vi "자판기 만들기 실습.vi"() -> ()   [LabVIEW 2020]
panel:
  in  "정지":bool
  in  "거스름돈 반환":bool
  out "배출 상품명":string
  out "현재잔액":dbl
  in  "1000원":bool
  in  "500원":bool
  in  "100원":bool
  in  "50원":bool
  in  "10원":bool
  out "웰치스 LED":bool
  out "콜라 LED":bool
  out "환타 LED":bool
  out "사이다 LED":bool
  in  "웰치스":bool
  in  "콜라":bool
  in  "환타":bool
  in  "사이다":bool
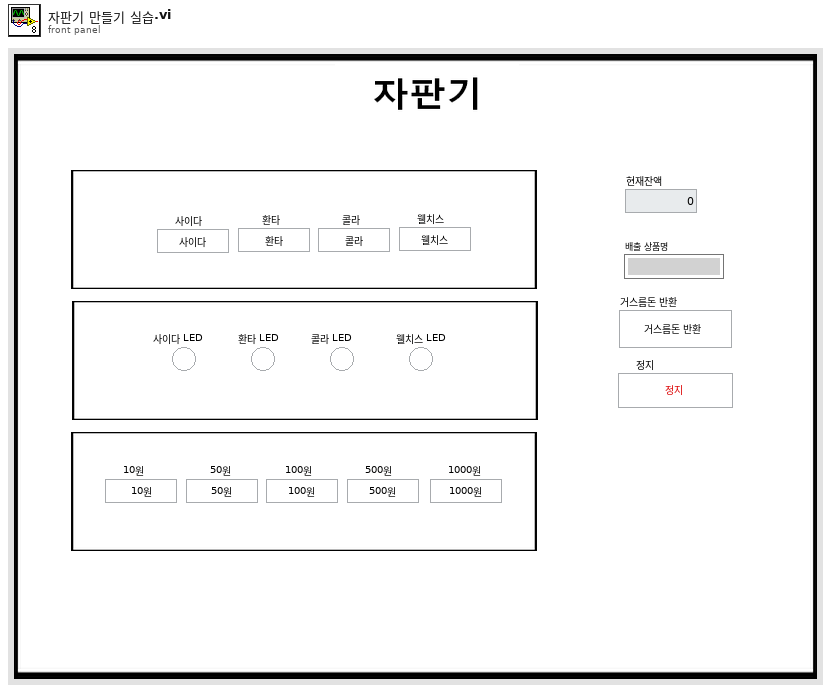
[diagram p1: front panel]
types:
  T1 = typedef "자판기 컨트롤.ctl" = enum16{"초기화", "대기", "10원", "50원", "100원", "500원", "1000원", "디스플레이 업데이트", "사이다", "콜라", "환타", "웰치스", "거스름돈 반환", "종료"}
  T2 = cluster{"상태":T1, "사이다 LED":bool, "현재잔액":dbl, "웰치스 LED":bool, "환타 LED":bool, "콜라 LED":bool, "배출 상품명":string}
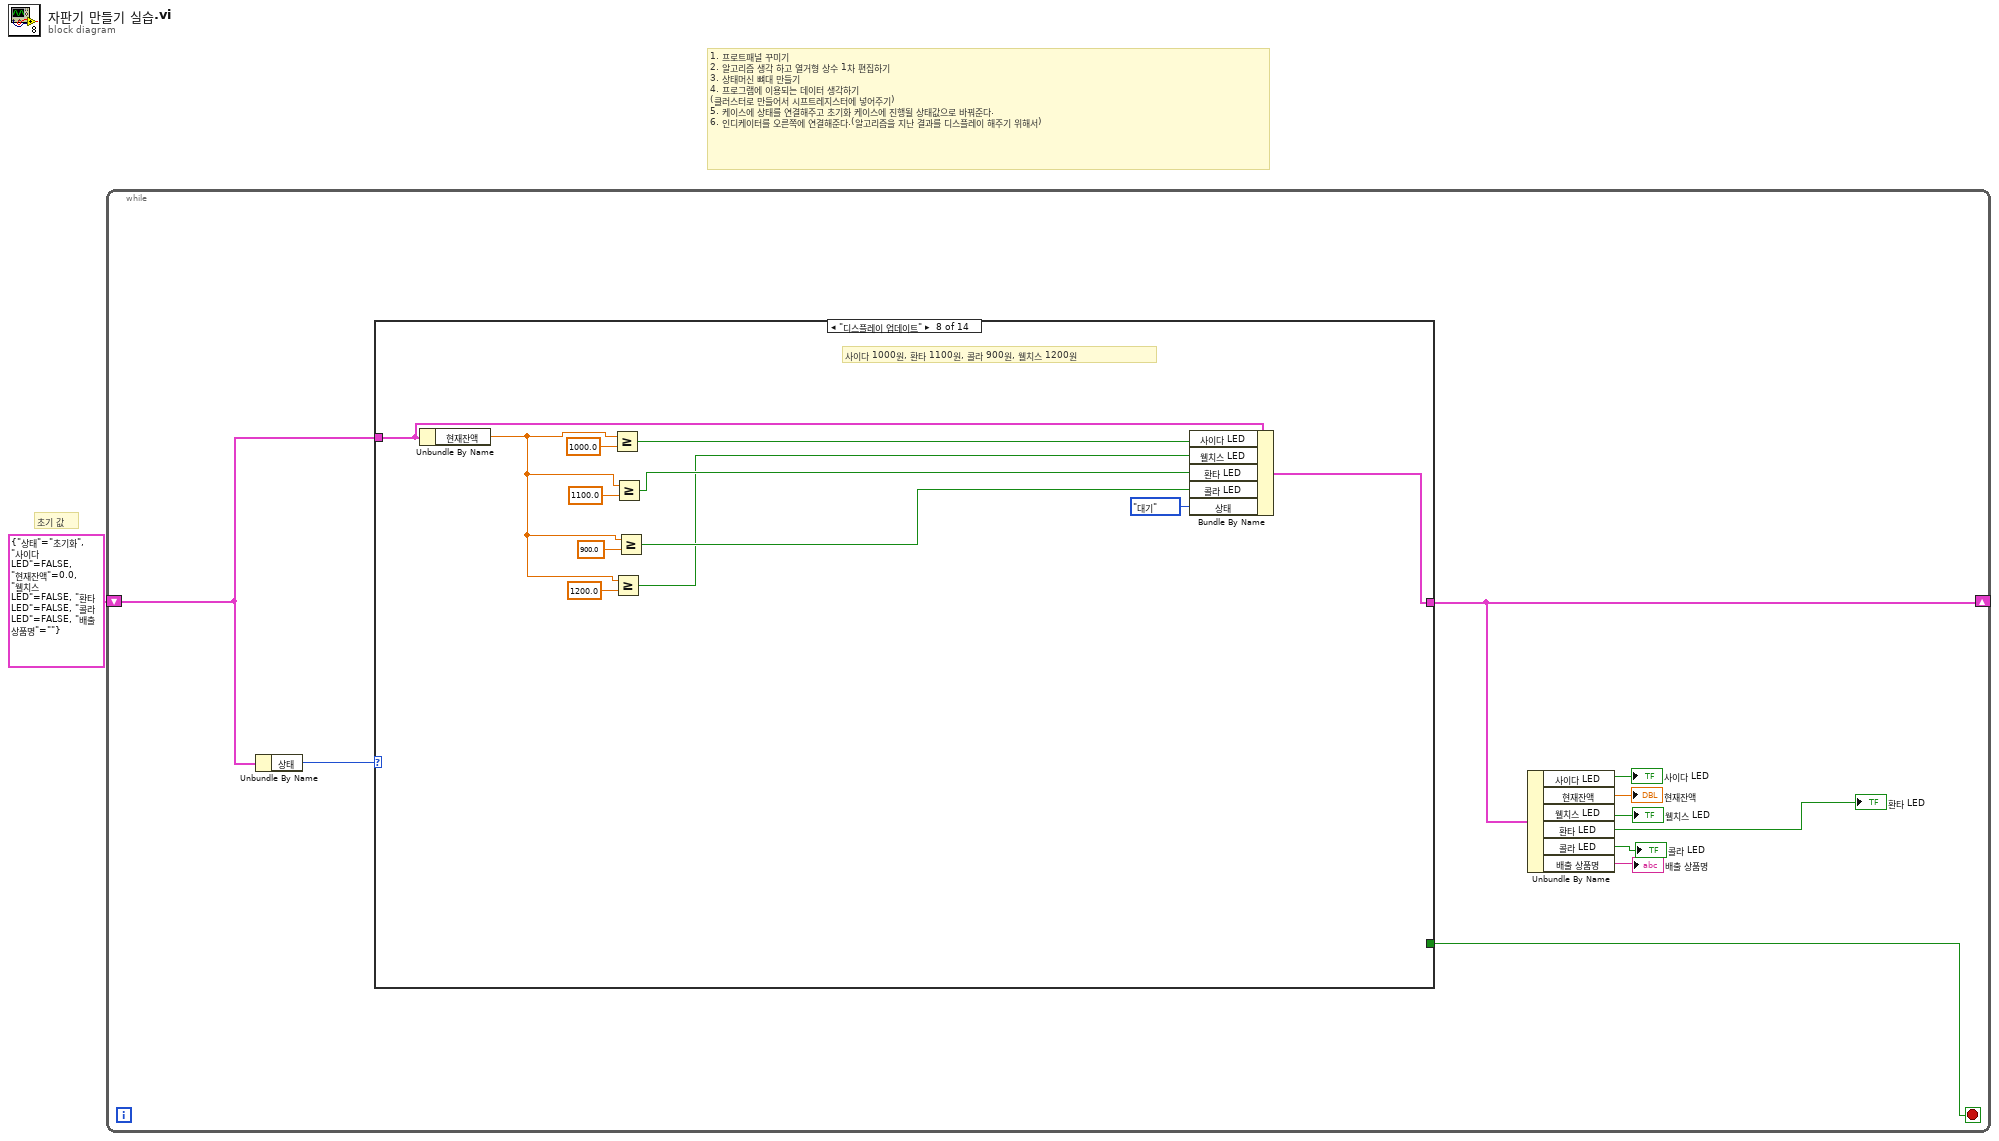
[diagram p0: block diagram]
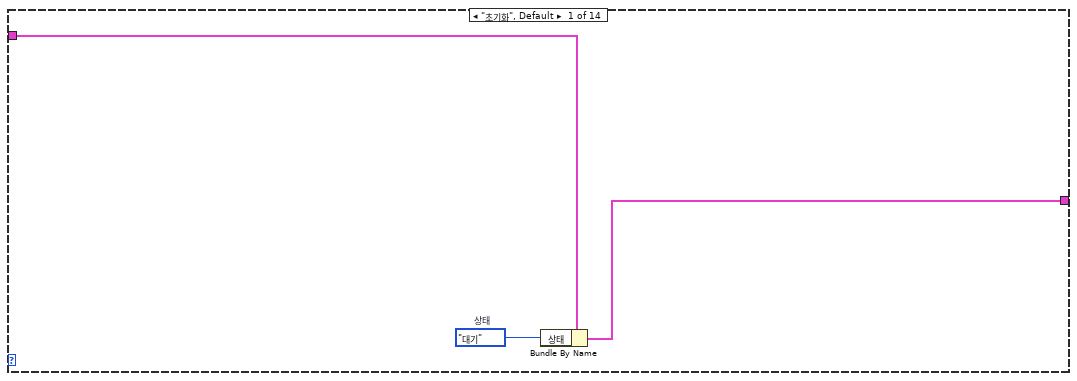
[diagram p2: hidden frame]
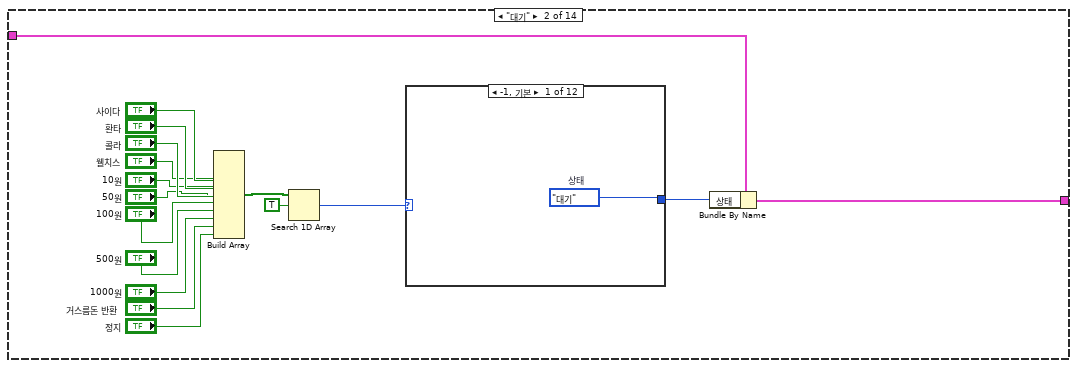
[diagram p3: hidden frame]
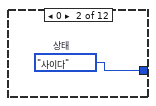
[diagram p4: hidden frame]
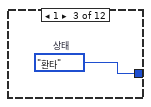
[diagram p5: hidden frame]
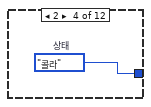
[diagram p6: hidden frame]
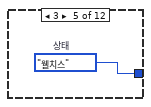
[diagram p7: hidden frame]
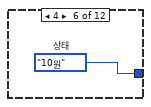
[diagram p8: hidden frame]
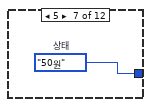
[diagram p9: hidden frame]
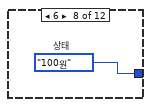
[diagram p10: hidden frame]
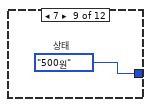
[diagram p11: hidden frame]
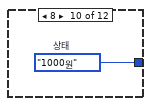
[diagram p12: hidden frame]
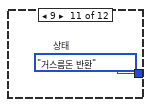
[diagram p13: hidden frame]
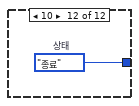
[diagram p14: hidden frame]
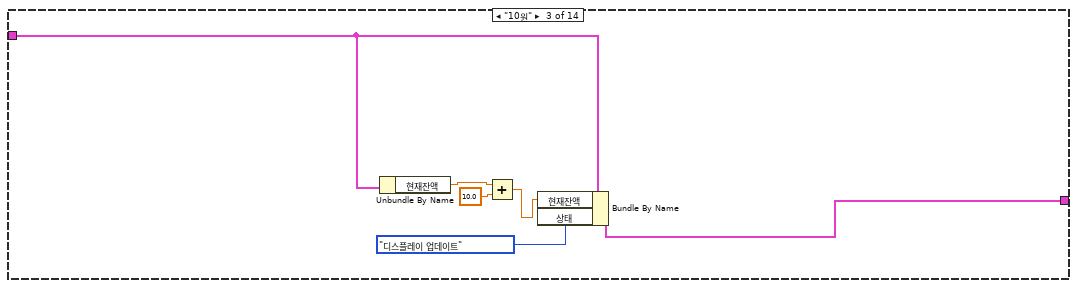
[diagram p15: hidden frame]
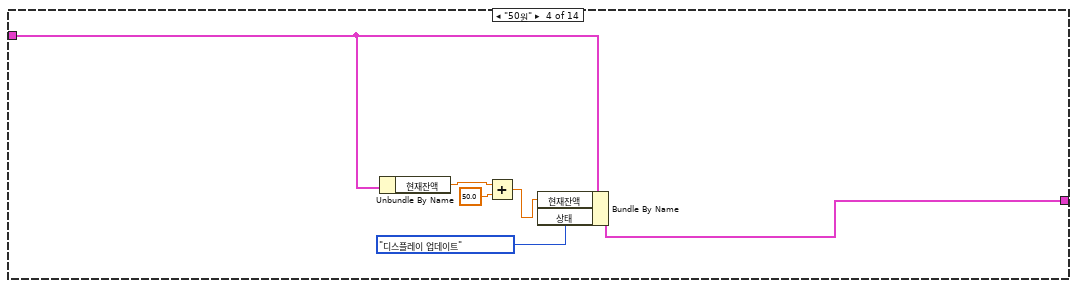
[diagram p16: hidden frame]
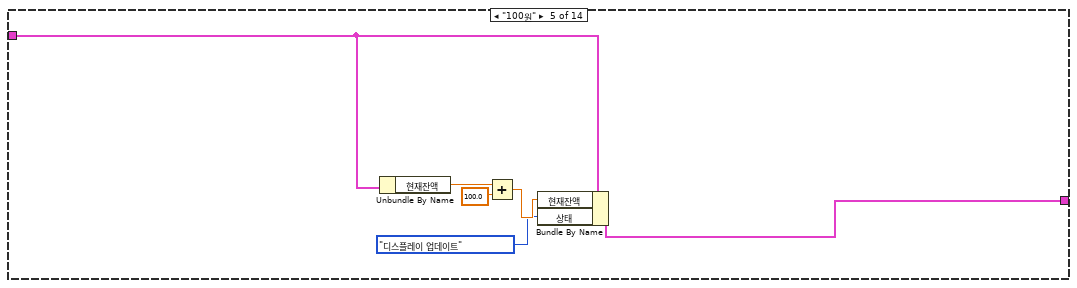
[diagram p17: hidden frame]
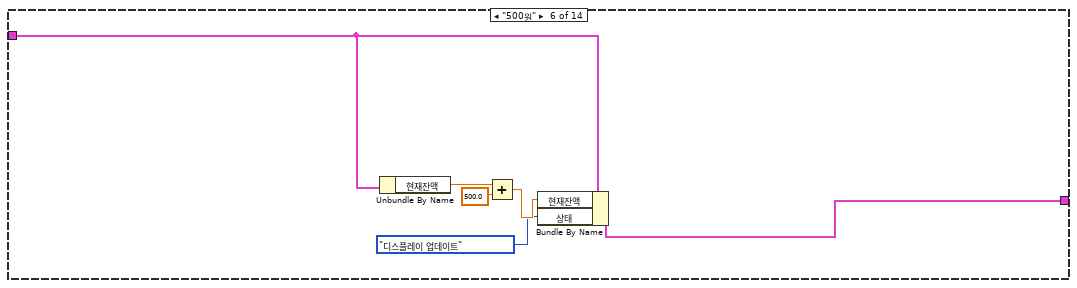
[diagram p18: hidden frame]
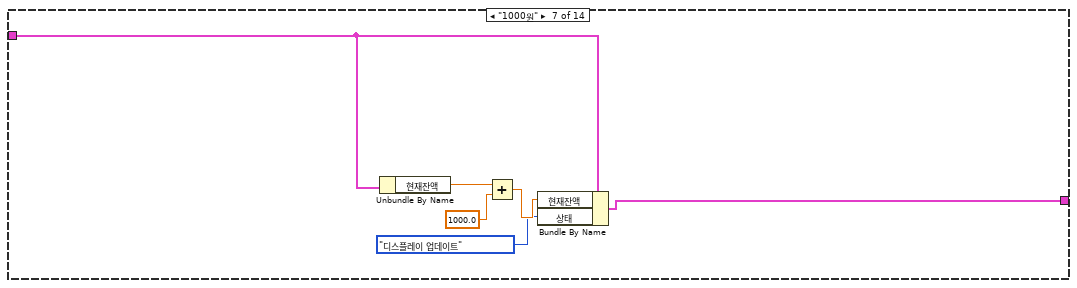
[diagram p19: hidden frame]
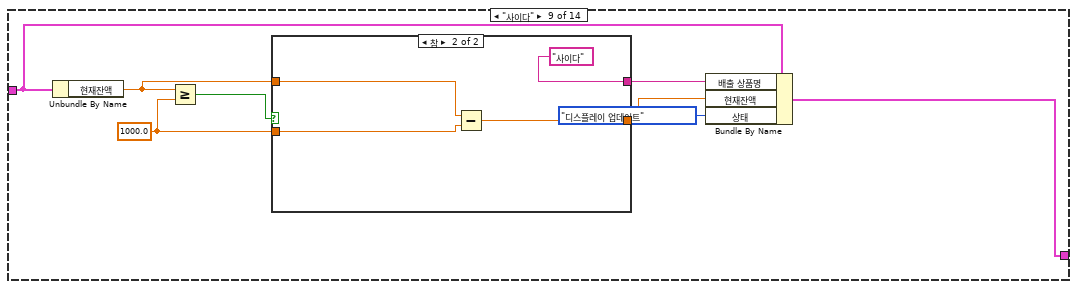
[diagram p20: hidden frame]
diagram:
  # "초기 값"
  # "1. 프로트패널 꾸미기\n2. 알고리즘 생각 하고 열거형 상수 1차 편집하기\n3. 상태머신 뼈대 만들기\n4. 프로그램에 이용되는 데이터 생각하기\n(클러스터로 만들어서 시프트레지스터에 넣어주기)\n5. 케이스에 상태를 연결해주고 초기화 케이스에 진행될 상태값으로 바꿔준다.\n6. 인디케이터를 오른쪽에 연결해준다.(알고리즘을 지난 결과를 디스플레이 해주기 위해서)"
  n1 = while {
    shift-right: [w9] -> _
    shift-left: T2 {"상태"=enum."초기화", "사이다 LED"=FALSE, "현재잔액"=0.0, "웰치스 LED"=FALSE, "환타 LED"=FALSE, "콜라 LED"=FALSE, "배출 상품명"=""} -> [w10]
    stop <- w5 stop-if-true
    n2 = Unbundle By Name(w10) -> ("상태"=w11:T1)
    n3 = case shown="\"디스플레이 업데이트\"" w11 {
      tunnel: w10 -> [w14 w17 w47 w53 w59 w65 w71 w84 w92 w106 w120 w134 w146 _]
      tunnel: [w12 w16 w45 w51 w57 w63 w69 w75 w90 w104 w118 w132 w145 _] -> w9
      tunnel: [_ _ _ _ _ _ _ _ _ _ _ _ _ TRUE] -> w5
      frame "초기화", Default {
        w13 = 자판기_컨트롤."대기"  # 상태
        n4 = Bundle By Name(cluster=w14, "상태"=w13) -> (w12:T2)
      }
      frame "대기" {
        n5 = Build Array("사이다", "환타", "콜라", "웰치스", "10원", "50원", "100원", "500원", "1000원", "거스름돈 반환", "정지") -> (w20:bool[])
        n6 = Search 1D Array(1D array=w20, element=TRUE ("원소")) -> (index of element=w18:i32)  [unwired: 1 in]
        n7 = case shown="-1, 기본" w18 {
          tunnel: [w32 w33 w34 w35 w36 w37 w38 w39 w40 w41 w42 w43] -> w15
          frame -1, Default {
            w32 = 자판기_컨트롤."대기"  # 상태
          }
          frame 0 {
            w33 = 자판기_컨트롤."사이다"  # 상태
          }
          frame 1 {
            w34 = 자판기_컨트롤."환타"  # 상태
          }
          frame 2 {
            w35 = 자판기_컨트롤."콜라"  # 상태
          }
          frame 3 {
            w36 = 자판기_컨트롤."웰치스"  # 상태
          }
          frame 4 {
            w37 = 자판기_컨트롤."10원"  # 상태
          }
          frame 5 {
            w38 = 자판기_컨트롤."50원"  # 상태
          }
          frame 6 {
            w39 = 자판기_컨트롤."100원"  # 상태
          }
          frame 7 {
            w40 = 자판기_컨트롤."500원"  # 상태
          }
          frame 8 {
            w41 = 자판기_컨트롤."1000원"  # 상태
          }
          frame 9 {
            w42 = 자판기_컨트롤."거스름돈 반환"  # 상태
          }
          frame 10 {
            w43 = 자판기_컨트롤."종료"  # 상태
          }
        }
        n8 = Bundle By Name(cluster=w17, "상태"=w15) -> (w16:T2)
      }
      frame "10원" {
        n9 = Unbundle By Name(w47) -> ("현재잔액"=w49:dbl)
        n10 = Add(x=w49, y=10.0) -> (x+y=w46:dbl)
        n11 = Bundle By Name(cluster=w47, "현재잔액"=w46, "상태"=자판기_컨트롤."디스플레이 업데이트") -> (w45:T2)
      }
      frame "50원" {
        n12 = Unbundle By Name(w53) -> ("현재잔액"=w55:dbl)
        n13 = Add(x=w55, y=50.0) -> (x+y=w52:dbl)
        n14 = Bundle By Name(cluster=w53, "현재잔액"=w52, "상태"=자판기_컨트롤."디스플레이 업데이트") -> (w51:T2)
      }
      frame "100원" {
        n15 = Unbundle By Name(w59) -> ("현재잔액"=w61:dbl)
        n16 = Add(x=w61, y=100.0) -> (x+y=w58:dbl)
        n17 = Bundle By Name(cluster=w59, "현재잔액"=w58, "상태"=자판기_컨트롤."디스플레이 업데이트") -> (w57:T2)
      }
      frame "500원" {
        n18 = Unbundle By Name(w65) -> ("현재잔액"=w67:dbl)
        n19 = Add(x=w67, y=500.0) -> (x+y=w64:dbl)
        n20 = Bundle By Name(cluster=w65, "현재잔액"=w64, "상태"=자판기_컨트롤."디스플레이 업데이트") -> (w63:T2)
      }
      frame "1000원" {
        n21 = Unbundle By Name(w71) -> ("현재잔액"=w73:dbl)
        n22 = Add(x=w73, y=1000.0) -> (x+y=w70:dbl)
        n23 = Bundle By Name(cluster=w71, "현재잔액"=w70, "상태"=자판기_컨트롤."디스플레이 업데이트") -> (w69:T2)
      }
      frame "디스플레이 업데이트" {
        # "사이다 1000원, 환타 1100원, 콜라 900원, 웰치스 1200원"
        n24 = Unbundle By Name(w84) -> ("현재잔액"=w77:dbl)
        n25 = Greater Or Equal?(x=w77, y=1000.0) -> (x >= y?=w83:bool)
        n26 = Greater Or Equal?(x=w77, y=1200.0) -> (x >= y?=w76:bool)
        n27 = Greater Or Equal?(x=w77, y=1100.0) -> (x >= y?=w81:bool)
        n28 = Greater Or Equal?(x=w77, y=900.0) -> (x >= y?=w79:bool)
        n29 = Bundle By Name(cluster=w84, "사이다 LED"=w83, "웰치스 LED"=w76, "환타 LED"=w81, "콜라 LED"=w79, "상태"=자판기_컨트롤."대기") -> (w75:T2)
      }
      frame "사이다" {
        w88 = 1000.0 ("y")
        n30 = Unbundle By Name(w92) -> ("현재잔액"=w89:dbl)
        n31 = Greater Or Equal?(x=w89, y=w88) -> (x >= y?=w93:bool)
        n32 = case shown="참" w93 {
          tunnel: ["잔액 부족" "사이다"] -> w91
          tunnel: w89 -> [w94 w98]
          tunnel: w88 -> [_ w97]
          tunnel: [w94 w96] -> w87
          frame False {
          }
          frame True {
            n33 = Subtract(x=w98, y=w97) -> (x-y=w96:dbl)
          }
        }
        n34 = Bundle By Name(cluster=w92, "배출 상품명"=w91, "현재잔액"=w87, "상태"=자판기_컨트롤."디스플레이 업데이트") -> (w90:T2)
      }
      frame "콜라" {
        w102 = 900.0 ("y")
        n35 = Unbundle By Name(w106) -> ("현재잔액"=w103:dbl)
        n36 = Greater Or Equal?(x=w103, y=w102) -> (x >= y?=w107:bool)
        n37 = case shown="참" w107 {
          tunnel: ["잔액 부족" "콜라"] -> w105
          tunnel: w103 -> [w108 w112]
          tunnel: w102 -> [_ w111]
          tunnel: [w108 w110] -> w101
          frame False {
          }
          frame True {
            n38 = Subtract(x=w112, y=w111) -> (x-y=w110:dbl)
          }
        }
        n39 = Bundle By Name(cluster=w106, "배출 상품명"=w105, "현재잔액"=w101, "상태"=자판기_컨트롤."디스플레이 업데이트") -> (w104:T2)
      }
      frame "환타" {
        w116 = 1100.0 ("y")
        n40 = Unbundle By Name(w120) -> ("현재잔액"=w117:dbl)
        n41 = Greater Or Equal?(x=w117, y=w116) -> (x >= y?=w121:bool)
        n42 = case shown="참" w121 {
          tunnel: ["잔액 부족" "환타"] -> w119
          tunnel: w117 -> [w122 w126]
          tunnel: w116 -> [_ w125]
          tunnel: [w122 w124] -> w115
          frame False {
          }
          frame True {
            n43 = Subtract(x=w126, y=w125) -> (x-y=w124:dbl)
          }
        }
        n44 = Bundle By Name(cluster=w120, "배출 상품명"=w119, "현재잔액"=w115, "상태"=자판기_컨트롤."디스플레이 업데이트") -> (w118:T2)
      }
      frame "웰치스" {
        w130 = 1200.0 ("y")
        n45 = Unbundle By Name(w134) -> ("현재잔액"=w131:dbl)
        n46 = Greater Or Equal?(x=w131, y=w130) -> (x >= y?=w135:bool)
        n47 = case shown="참" w135 {
          tunnel: ["잔액 부족" "웰치스"] -> w133
          tunnel: w131 -> [w136 w140]
          tunnel: w130 -> [_ w139]
          tunnel: [w136 w138] -> w129
          frame False {
          }
          frame True {
            n48 = Subtract(x=w140, y=w139) -> (x-y=w138:dbl)
          }
        }
        n49 = Bundle By Name(cluster=w134, "배출 상품명"=w133, "현재잔액"=w129, "상태"=자판기_컨트롤."디스플레이 업데이트") -> (w132:T2)
      }
      frame "거스름돈 반환" {
        n50 = Bundle By Name(cluster=w146, "현재잔액"=0.0, "배출 상품명"="잔액반환", "상태"=자판기_컨트롤."디스플레이 업데이트") -> (w145:T2)
      }
      frame "종료" {
      }
    }
    n51 = Unbundle By Name(w9) -> ("사이다 LED"=→"사이다 LED":bool, "현재잔액"=→"현재잔액":dbl, "웰치스 LED"=→"웰치스 LED":bool, "환타 LED"=→"환타 LED":bool, "콜라 LED"=→"콜라 LED":bool, "배출 상품명"=→"배출 상품명":string)
  }
